vi "VersionController.vi"() -> ()   [LabVIEW 2019, in "ByteLVDevEnv.lvlib"]
uses:
  ByteLVDevEnv.lvlib
  TypeDefs/LibraryVersions.ctl
  TypeDefs/AllLibraries.ctl
  <vilib>/regexp/Match Regular Expression.xnode
  <vilib>/JKI/VIPM API/VIPM API_vipm_api.lvlib
panel:
  in  "Select Labview Version":u16(ring) items=["19.0"]
  out "Status":string
  in  "Exit":bool
  in  "Restart":bool
  out "LOADING":string
  out "packets.txt errors":string[](array[string])
  in  "Local VIP Folder":path
  out "VIP files found in local folder":string
  out "Install log":string[](array[string])
  in  "Start":bool
  in  "packets.txt Path":path
  # "VIP Package Installer"
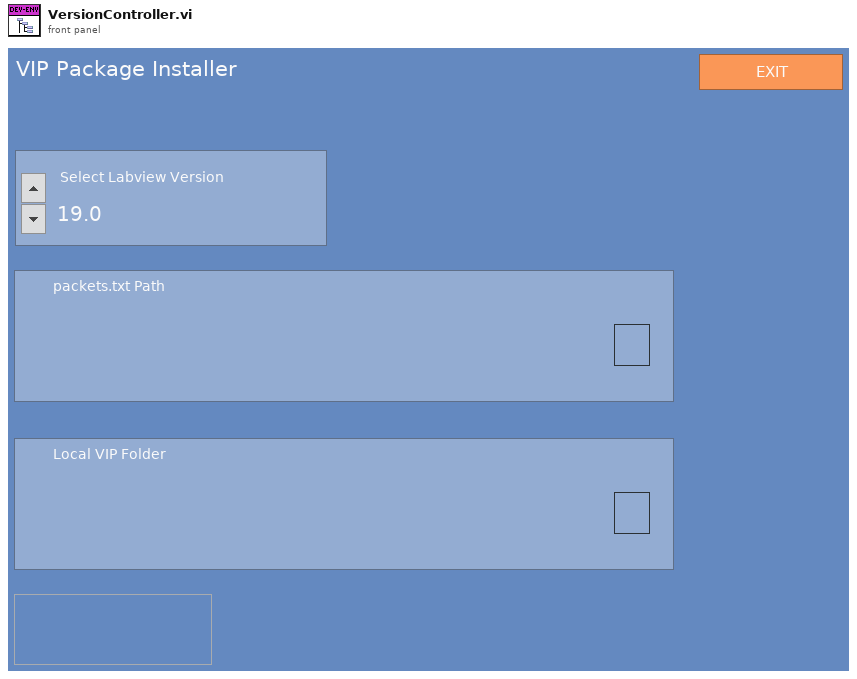
[diagram p1: front panel]
types:
  T1 = typedef "ByteLVDevEnv.lvlib/AllLibraries.ctl" = cluster{"Package Name":string, "Version":string, "Installed":bool, "Path":path}
  T2 = typedef "ByteLVDevEnv.lvlib/LibraryVersions.ctl" = cluster{"Name":string, "Version 1 ":string, "Version 2":string, "Sign 1":string, "Sign 2":string, "Function":string, "V. Install":string}
  T3 = cluster{"LOADING":refnum<vi>, "Local VIP Folder":refnum<vi>, "packets.txt Path ":refnum<vi>, "Start":refnum<vi>, "Install log":refnum<vi>, "VIP files found in local folder":refnum<vi>, "packets.txt errors":refnum<vi>, "Restart":refnum<vi>, "Exit":refnum<vi>, "Status":refnum<vi>, "Select Labview Version":refnum<vi>}
  T4 = cluster{"Status":string, "Versions":T2[], "All Packages":T1[], "LabView V.":string, "LocalVip":T1[], "Log":string[], "Packets errors":string[]}
  T5 = enum8{"Enabled", "Disabled", "Disabled and Grayed Out"}
  T6 = enum16{"open", "replace", "create", "open or create", "replace or create", "replace or create with confirmation"}
  T7 = cluster{"packets.txt Path ":path, "Local VIP Folder":path, "Select Labview Version":u16}
  T8 = typedef "VIPM API_vipm_api.lvlib/LabVIEW Target Info Cluster_vipm_api.ctl" = cluster{"Version":string, "Connection Tested":bool, "Disabled":bool}
  T9 = typedef "LVStringsAndValuesArrayTypeDef_U16.ctl" = cluster{"String":string, "Value":u16}[]
  T10 = typedef "VIPM API_vipm_api.lvlib/Library Contents Cluster_vipm_api.ctl" = cluster{"Package Name":string, "Version":string, "Display Name":string, "Repository Name":string, "Company Name":string, "License Type":string, "Installed":bool, "Deprecated":bool, "Dependency or Conflict Problem":bool, "Downloaded":bool}
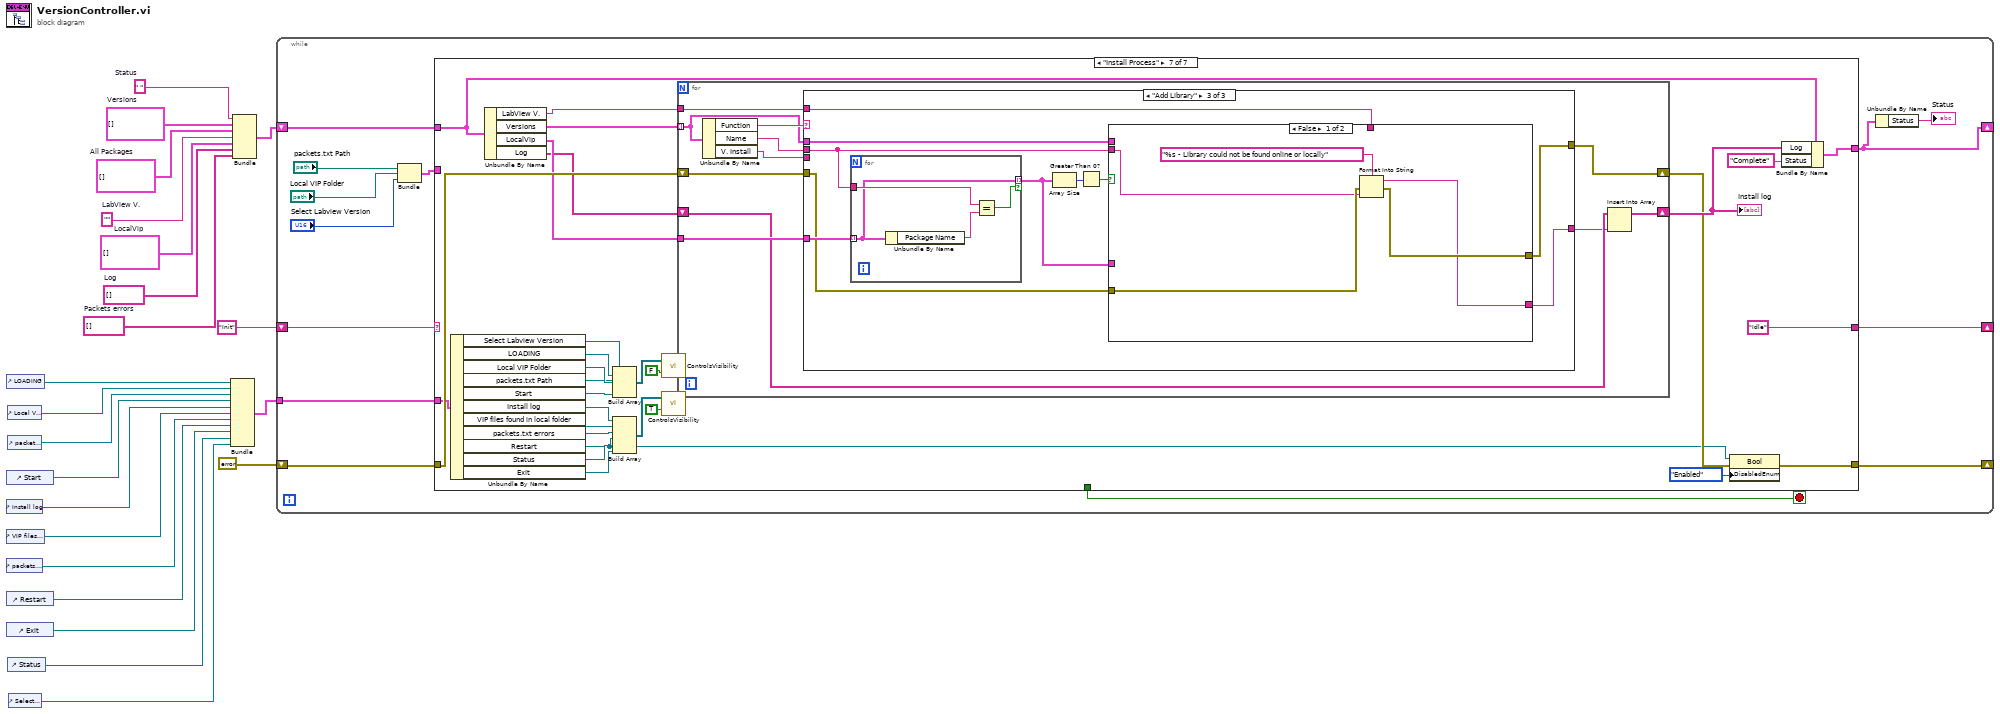
[diagram p0: block diagram]
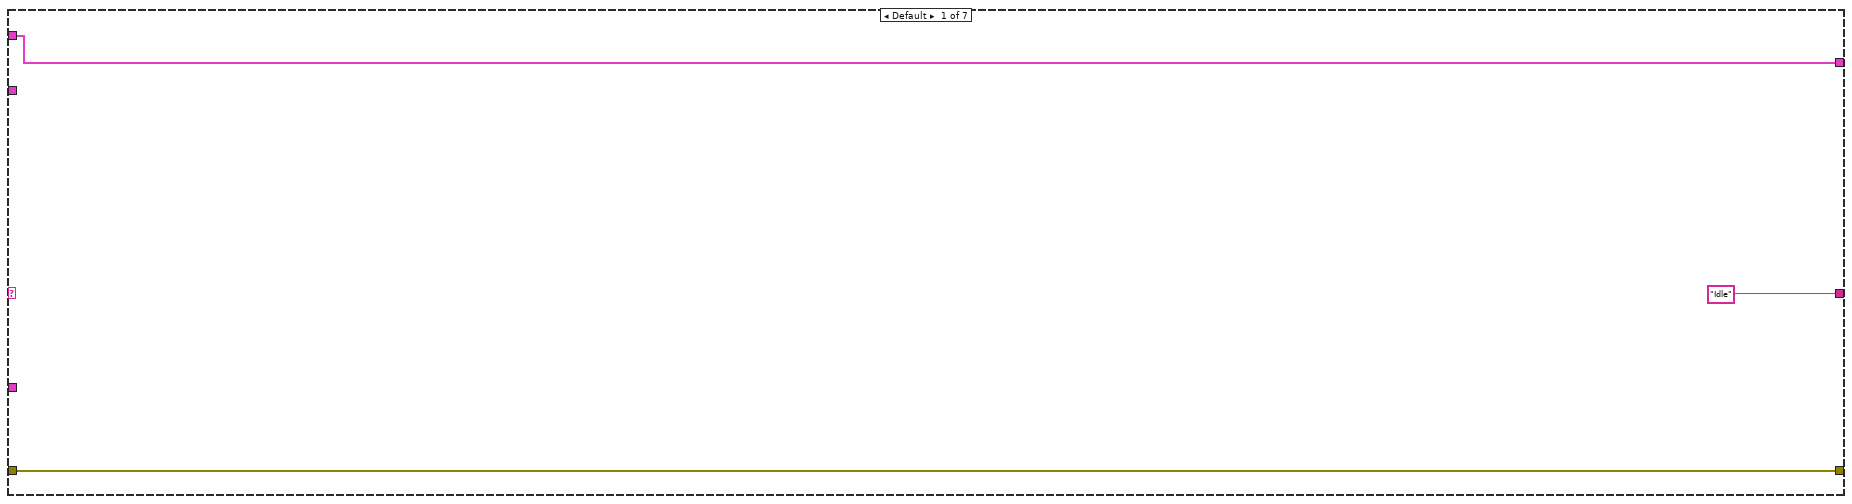
[diagram p2: hidden frame]
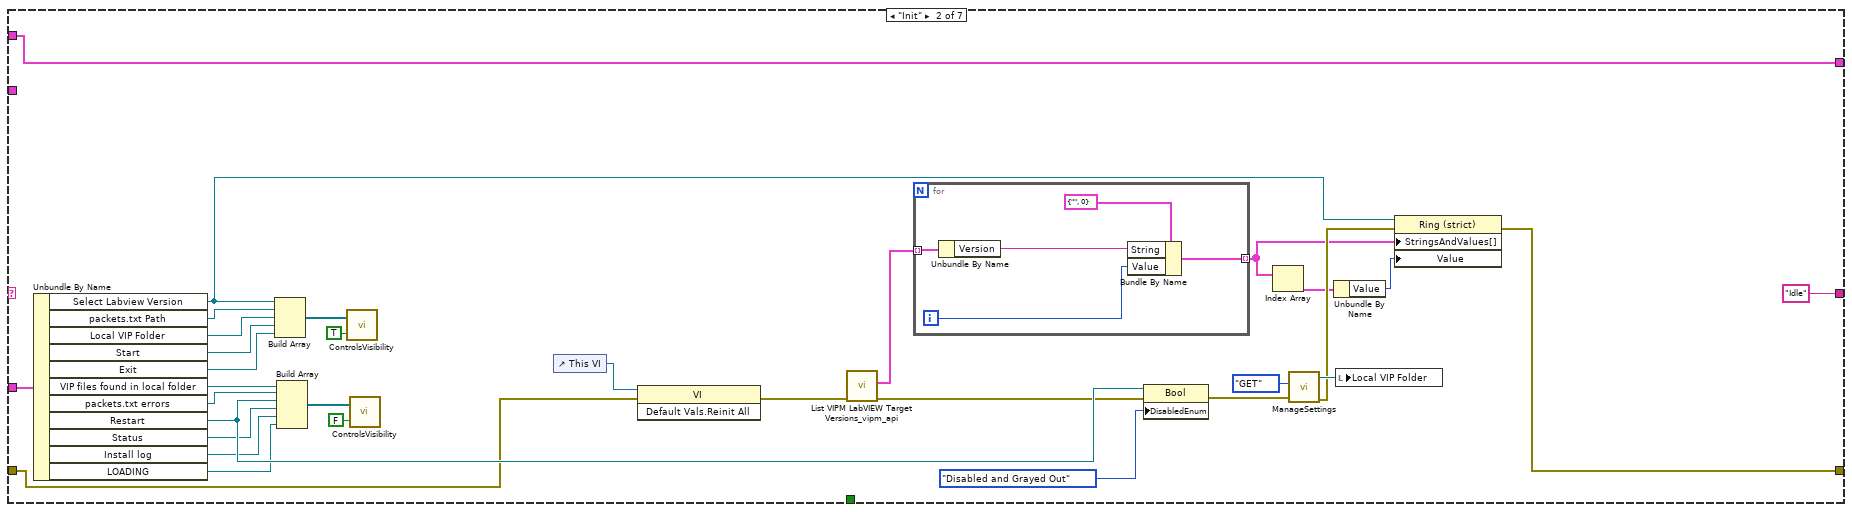
[diagram p3: hidden frame]
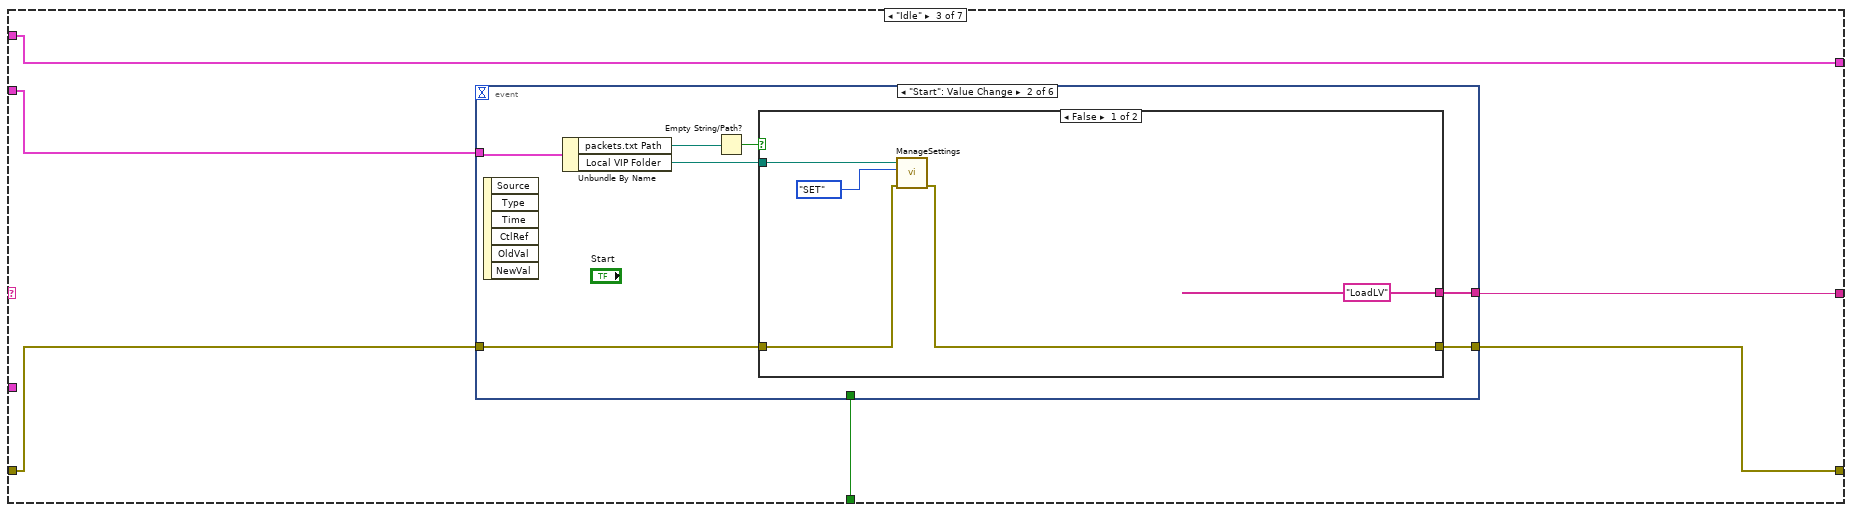
[diagram p4: hidden frame]
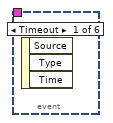
[diagram p5: hidden frame]
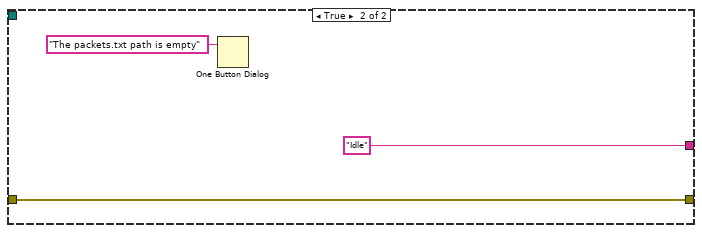
[diagram p6: hidden frame]
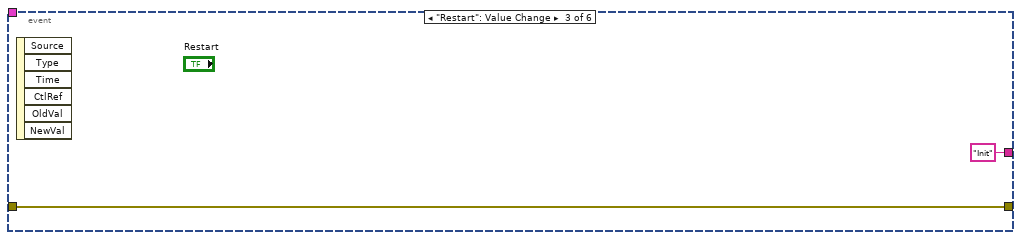
[diagram p7: hidden frame]
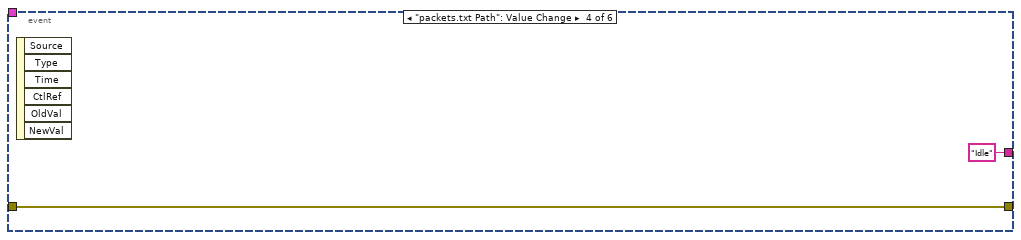
[diagram p8: hidden frame]
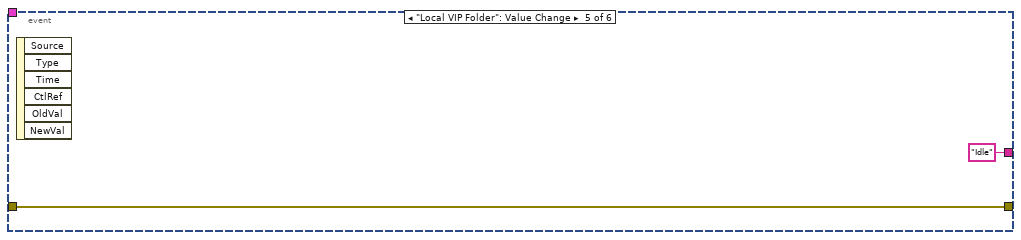
[diagram p9: hidden frame]
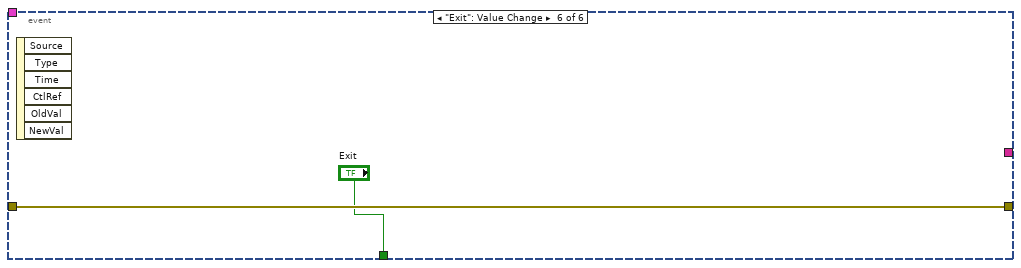
[diagram p10: hidden frame]
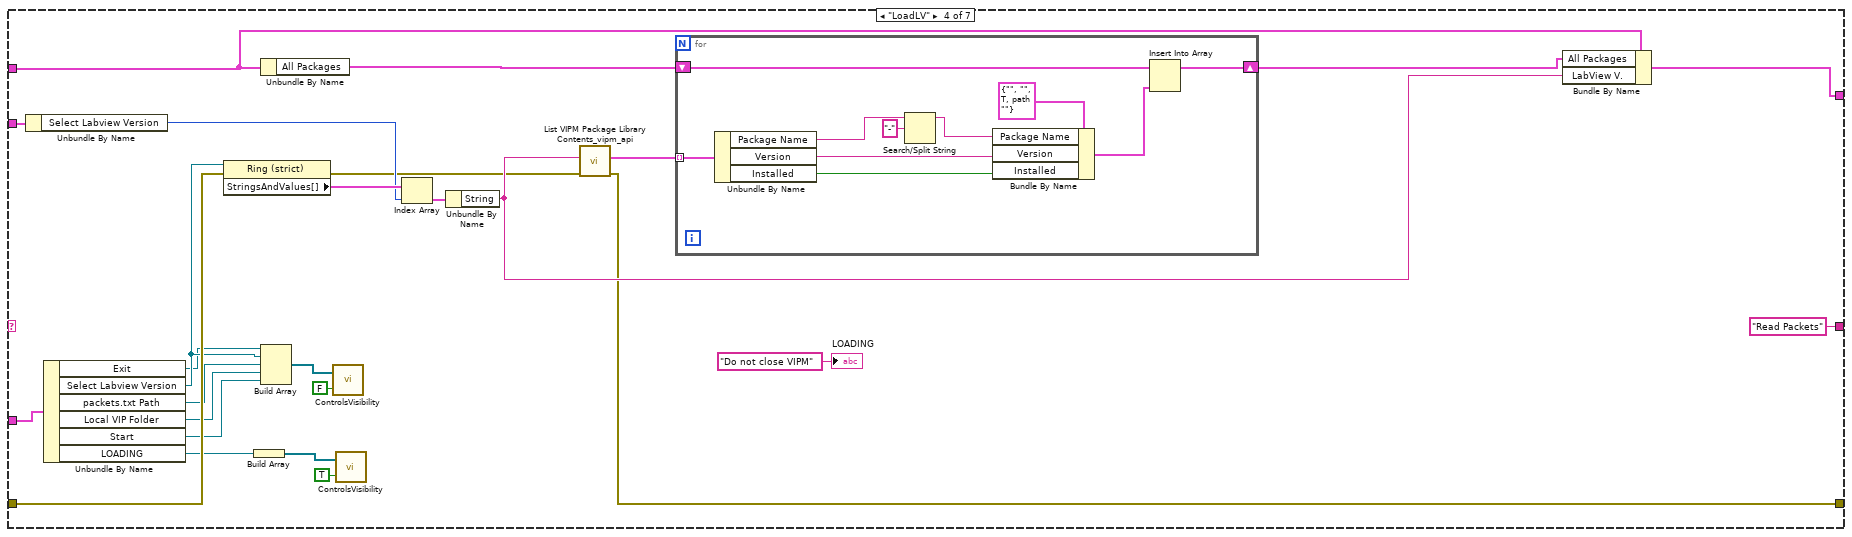
[diagram p11: hidden frame]
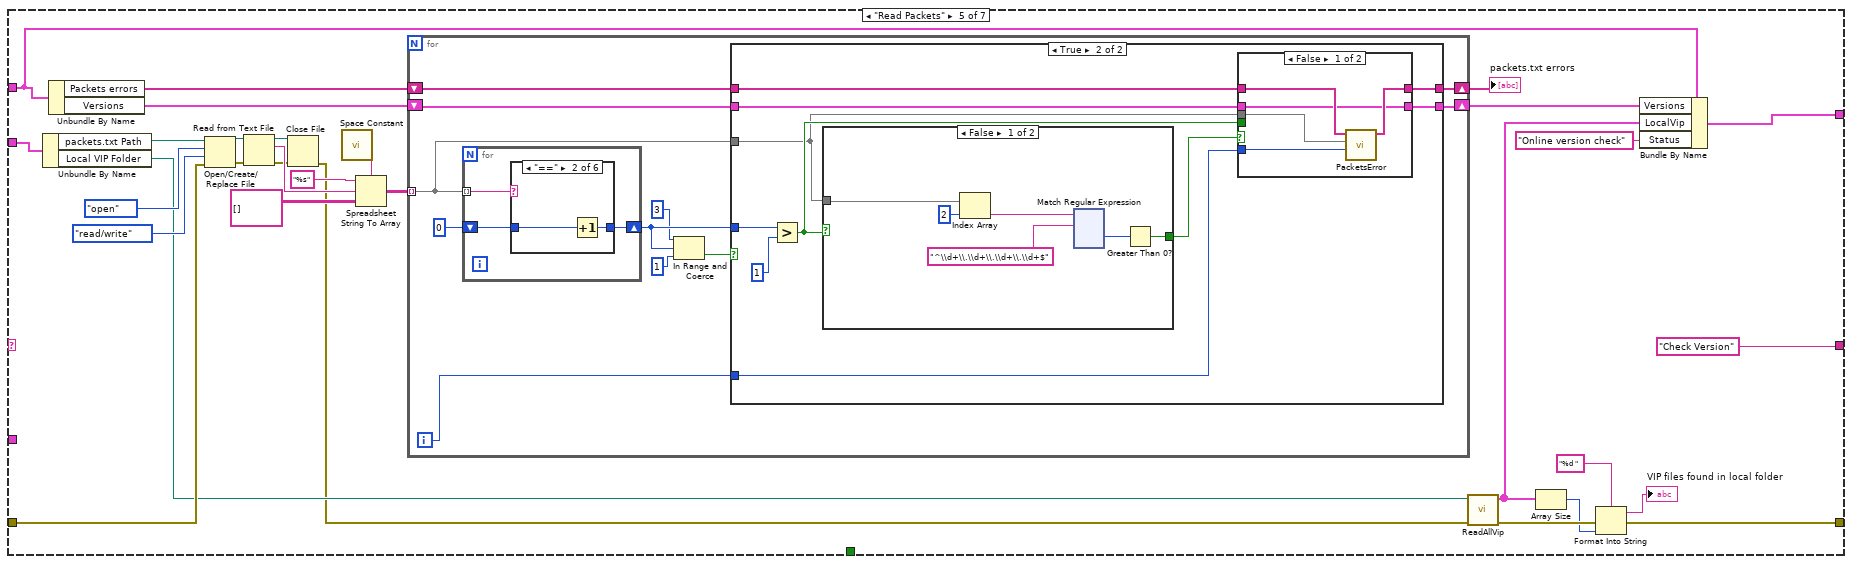
[diagram p12: hidden frame]
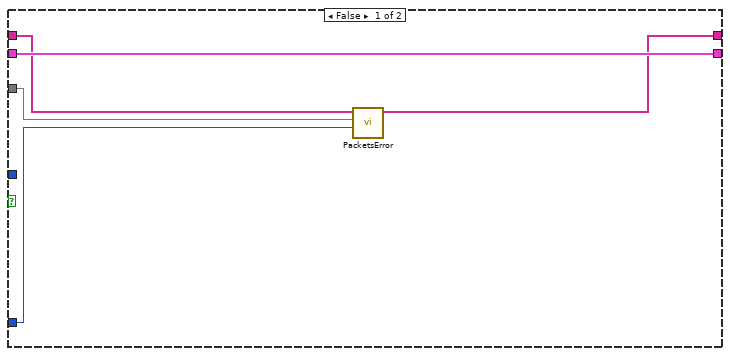
[diagram p13: hidden frame]
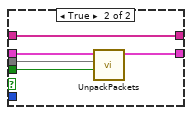
[diagram p14: hidden frame]
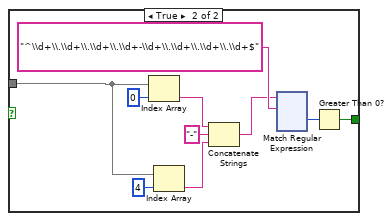
[diagram p15: hidden frame]
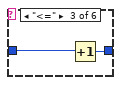
[diagram p17: hidden frame]
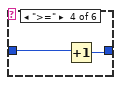
[diagram p18: hidden frame]
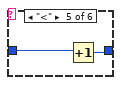
[diagram p19: hidden frame]
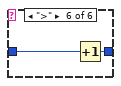
[diagram p20: hidden frame]
diagram:
  w3 = " "  # Status
  w14 = string[] []  # Packets errors
  w15 = string[] []  # Log
  w16 = T1[] []  # LocalVip
  w18 = ""  # LabView V.
  w19 = T1[] []  # All Packages
  w21 = T2[] []  # Versions
  n1 = control-ref of="LOADING"() -> (w13:refnum<vi>)
  n2 = control-ref of="Start"() -> (w10:refnum<vi>)
  n3 = control-ref of="Install log"() -> (w9:refnum<vi>)
  n4 = control-ref of="VIP files found in local folder"() -> (w8:refnum<vi>)
  n5 = control-ref of="packets.txt errors"() -> (w7:refnum<vi>)
  n6 = control-ref of="Restart"() -> (w5:refnum<vi>)
  n7 = control-ref of="Exit"() -> (w4:refnum<vi>)
  n8 = control-ref of="Local VIP Folder"() -> (w12:refnum<vi>)
  n9 = control-ref of="packets.txt Path"() -> (w11:refnum<vi>)
  n10 = control-ref of="Status"() -> (w2:refnum<vi>)
  n11 = control-ref of="Select Labview Version"() -> (w1:refnum<vi>)
  n12 = Bundle("LOADING"=w13, "Local VIP Folder"=w12, "packets.txt Path"=w11, "Start"=w10, "Install log"=w9, "VIP files found in local folder"=w8, "packets.txt errors"=w7, "Restart"=w5, "Exit"=w4, "Status"=w2, "Select Labview Version"=w1) -> (w6:T3)  [unwired: 1 in]
  n13 = Bundle("Status"=w3, "Versions"=w21, "All Packages"=w19, "LabView V."=w18, "LocalVip"=w16, "Log"=w15, "Packets errors"=w14) -> (w20:T4)  [unwired: 1 in]
  n14 = while {
    shift-right: [w32] -> _
    shift-left: "Init" -> [w35]
    shift-right: [w25] -> _
    shift-left: w20 -> [w31]
    shift-right: [w30] -> _
    shift-left: errorcluster {"status"=FALSE, "code"=0, "source"=""} ("error in") -> [w29]
    tunnel: w6 -> [w27]
    stop <- w26 stop-if-true
    n15 = Bundle("packets.txt Path"="packets.txt Path", "Local VIP Folder"="Local VIP Folder", "Select Labview Version"="Select Labview Version") -> (w33:T7)  [unwired: 1 in]
    n16 = case shown="\"Install Process\"" w35 {
      tunnel: w33 -> [_ _ w79 w122 w170 _ _]
      tunnel: ["Idle" "Idle" w81 "Read Packets" "Check Version" "Install Process" "Idle"] -> w32
      tunnel: w31 -> [w37 w69 w80 w128 w157 w469 w519]
      tunnel: w29 -> [w36 w48 w78 w124 w168 w470 w523]
      tunnel: [w37 w69 w80 w127 w155 w466 w518] -> w25
      tunnel: [w36 w43 w77 w107 w148 w470 w502] -> w30
      tunnel: w27 -> [_ w65 _ w125 _ _ w506]
      tunnel: [_ _ w76 _ _ _ _] -> w26
      frame Default {
      }
      frame "Init" {
        n17 = Unbundle By Name(w65) -> ("Select Labview Version"=w42:refnum<vi>, "packets.txt Path"=w60:refnum<vi>, "Local VIP Folder"=w59:refnum<vi>, "Start"=w58:refnum<vi>, "Exit"=w57:refnum<vi>, "VIP files found in local folder"=w56:refnum<vi>, "packets.txt errors"=w55:refnum<vi>, "Restart"=w54:refnum<vi>, "Status"=w53:refnum<vi>, "Install log"=w52:refnum<vi>, "LOADING"=w51:refnum<vi>)
        n18 = Build Array(w42, w60, w59, w58, w57) -> (w49:refnum<vi>[])
        n19 = Build Array(w56, w55, w54, w53, w52, w51) -> (w50:refnum<vi>[])
        n20 = call "ControlsVisibility.vi"("Visible"=TRUE, "Array"=w49) -> ()  [unwired: 2 in]
        n21 = call "ControlsVisibility.vi"("Visible"=FALSE, "Array"=w50) -> ()  [unwired: 2 in]
        n22 = control-ref of="This VI"() -> (w67:refnum<vi>)
        n23 = invoke class="VI" method="Default Vals.Reinit All"(reference=w67, error in=w48) -> (error out=w47:errorcluster)  [unwired: 1 in, 2 out]
        n24 = call <vilib>:"List VIPM LabVIEW Target Versions_vipm_api.vi"("error in (no error)"=w47) -> ("error out"=w46:errorcluster, "LabVIEW Target Info"=w45:T8[])  [unwired: 9 in]
        n25 = for {
          tunnel: w45 -> [w74] mode=indexing
          tunnel: [w71] -> w41 mode=indexing
          i -> [w72]
          n26 = Unbundle By Name(w74) -> ("Version"=w73:string)
          n27 = Bundle By Name(cluster=cluster{"String":string, "Value":u16} {"String"="", "Value"=0} ("Cluster"), "String"=w73, "Value"=w72) -> (w71:cluster{"String":string, "Value":u16})
        }
        n28 = property class="Bool"(reference=w54, error in=w46, "DisabledEnum"=T5."Disabled and Grayed Out" ("Disabled")) -> (error out=w63:errorcluster)  [unwired: 1 out]
        n29 = Index Array(array=w41) -> (element=w40:cluster{"String":string, "Value":u16})  [unwired: 1 in]
        n30 = call "ManageSettings.vi"("error in (no error)"=w63, "Mode"=enum16{"GET", "SET"}."GET") -> ("error out"=w44:errorcluster, "File Path Out"=w66:path)  [unwired: 8 in]
        n31 = Unbundle By Name(w40) -> ("Value"=w39:u16)
        n32 = local write "Local VIP Folder"(w66) -> ()
        n33 = property class="Ring (strict)"(reference=w42, error in=w44, "StringsAndValues[]"=w41, "Value"=w39) -> (error out=w43:errorcluster)  [unwired: 1 out]
      }
      frame "Idle" {
        n34 = event shown="[1] \"Start\": Value Change" {
          selector: _ -> [_ _ _ _ _ _]
          dyn-events: _ -> [_ _ _ _ _ _]
          timeout: _ -> [_ _ _ _ _ _]
          tunnel: [_ w85 "Init" "Idle" "Idle" _] -> w81
          tunnel: w79 -> [_ w88 _ _ _ _]
          tunnel: w78 -> [_ w83 w98 w99 w101 w104]
          tunnel: [_ w82 w98 w99 w101 w104] -> w77
          tunnel: [_ _ _ _ _ "Exit"] -> w76
          event Timeout {
            n35 = event-data() -> ()  [unwired: 1 in, 3 out]
          }
          event "Start": Value Change {
            n36 = event-data() -> ()  [unwired: 1 in, 6 out]
            n37 = Unbundle By Name(w88) -> ("packets.txt Path"=w87:path, "Local VIP Folder"=w84:path)
            n38 = Empty String/Path?(string/path=w87) -> (empty?=w86:bool)
            n39 = case shown="False" w86 {
              tunnel: ["LoadLV" "Idle"] -> w85
              tunnel: w84 -> [w92 _]
              tunnel: w83 -> [w90 w95]
              tunnel: [w89 w95] -> w82
              frame False {
                n40 = call "ManageSettings.vi"("error in (no error)"=w90, "Mode"=enum16{"GET", "SET"}."SET", "File Path"=w92) -> ("error out"=w89:errorcluster)  [unwired: 7 in, 1 out]
              }
              frame True {
                n41 = One Button Dialog(message="The packets.txt path is empty") -> ()  [unwired: 1 in, 1 out]
              }
            }
          }
          event "Restart": Value Change {
            n42 = event-data() -> ()  [unwired: 1 in, 6 out]
          }
          event "packets.txt Path": Value Change {
            n43 = event-data() -> ()  [unwired: 1 in, 6 out]
          }
          event "Local VIP Folder": Value Change {
            n44 = event-data() -> ()  [unwired: 1 in, 6 out]
          }
          event "Exit": Value Change {
            n45 = event-data() -> ()  [unwired: 1 in, 6 out]
          }
        }
      }
      frame "LoadLV" {
        n46 = Unbundle By Name(w122) -> ("Select Labview Version"=w121:u16)
        n47 = Unbundle By Name(w125) -> ("Exit"=w105:refnum<vi>, "Select Labview Version"=w112:refnum<vi>, "packets.txt Path"=w111:refnum<vi>, "Local VIP Folder"=w110:refnum<vi>, "Start"=w109:refnum<vi>, "LOADING"=w108:refnum<vi>)
        n48 = property class="Ring (strict)"(reference=w112, error in=w124) -> (error out=w117:errorcluster, "StringsAndValues[]"=w123:T9)  [unwired: 1 out]
        n49 = Build Array(w108) -> (w114:refnum<vi>[])
        n50 = Unbundle By Name(w128) -> ("All Packages"=w130:T1[])
        n51 = Build Array(w105, w112, w111, w110, w109) -> (w113:refnum<vi>[])
        n52 = call "ControlsVisibility.vi"("Visible"=FALSE, "Array"=w113) -> ()  [unwired: 2 in]
        n53 = call "ControlsVisibility.vi"("Visible"=TRUE, "Array"=w114) -> ()  [unwired: 2 in]
        n54 = Index Array(array=w123, index=w121) -> (element=w120:cluster{"String":string, "Value":u16})
        n55 = Unbundle By Name(w120) -> ("String"=w119:string)
        n56 = call <vilib>:"List VIPM Package Library Contents_vipm_api.vi"("error in (no error)"=w117, "LabVIEW Version"=w119) -> ("error out"=w107:errorcluster, "Library Contents []"=w129:T10[])  [unwired: 7 in, 1 out]
        n57 = for {
          tunnel: w129 -> [w140] mode=indexing
          shift-right: [w133] -> w126
          shift-left: w130 -> [w132]
          n58 = Unbundle By Name(w140) -> ("Package Name"=w138:string, "Version"=w135:string, "Installed"=w134:bool)
          n59 = Search/Split String(string=w138, search string/char (-)="-") -> (substring before match=w136:string)  [unwired: 1 in, 2 out]
          n60 = Bundle By Name(cluster=T1 {"Package Name"="", "Version"="", "Installed"=TRUE, "Path"=path ""}, "Package Name"=w136, "Version"=w135, "Installed"=w134) -> (w131:T1)
          n61 = Insert Into Array(array=w132, new element=w131) -> (w133:T1[])  [unwired: 1 in]
        }
        n62 = Bundle By Name(cluster=w128, "All Packages"=w126, "LabView V."=w119) -> (w127:T4)
        "LOADING" <- "Do not close VIPM" ("LOADING")
      }
      frame "Read Packets" {
        n63 = Unbundle By Name(w170) -> ("packets.txt Path"=w169:path, "Local VIP Folder"=w153:path)
        n64 = Unbundle By Name(w157) -> ("Packets errors"=w146:string[], "Versions"=w158:T2[])
        n65 = Open/Create/Replace File(file path (use dialog)=w169, error in=w168, operation (0:open)=T6."open", access (0:read/write)=enum16{"read/write", "read-only", "write-only"}."read/write") -> (refnum out=w165:refnum<file>, error out=w164:errorcluster)  [unwired: 2 in, 1 out]
        n66 = Read from Text File(file (use dialog)=w165, error in=w164) -> (refnum out=w142:refnum<file>, text=w163:string, error out=w143:errorcluster)  [unwired: 2 in, 1 out]
        n67 = Close File(refnum=w142, error in=w143) -> (error out=w141:errorcluster)  [unwired: 1 out]
        n68 = call <vilib>:"Space Constant.vi"() -> ("String"=w159:string)
        n69 = Spreadsheet String To Array(delimiter (Tab)=w159, format string="%s", spreadsheet string=w163, array type (2D Dbl)=string[][] []) -> (array=w160:string[][])
        n70 = for {
          tunnel: w160 -> [w178] mode=indexing
          shift-right: [w180] -> w156
          shift-left: w158 -> [w181]
          shift-right: [w172] -> w145
          shift-left: w146 -> [w173]
          i -> [w171]
          n71 = for {
            tunnel: w178 -> [w453] mode=indexing
            shift-right: [w451] -> w177
            shift-left: 0 -> [w452]
            n72 = case shown="\"==\"" w453 {
              tunnel: w452 -> [w454 w456 w458 w460 w462 w464]
              tunnel: [w454 w455 w457 w459 w461 w463] -> w451
              frame Default {
              }
              frame "==" {
                n73 = Increment(x=w456) -> (x+1=w455:i32)
              }
              frame "<=" {
                n74 = Increment(x=w458) -> (x+1=w457:i32)
              }
              frame ">=" {
                n75 = Increment(x=w460) -> (x+1=w459:i32)
              }
              frame "<" {
                n76 = Increment(x=w462) -> (x+1=w461:i32)
              }
              frame ">" {
                n77 = Increment(x=w464) -> (x+1=w463:i32)
              }
            }
          }
          n78 = In Range and Coerce(upper limit=3, x=w177, lower limit=1) -> (In Range?=w174:bool)  [unwired: 1 out]
          n79 = case shown="True" w174 {
            tunnel: w181 -> [w186 w196]
            tunnel: [w186 w195] -> w180
            tunnel: w178 -> [w185 w191]
            tunnel: w177 -> [_ w193]
            tunnel: w173 -> [w184 w190]
            tunnel: [w183 w189] -> w172
            tunnel: w171 -> [w182 w188]
            frame False {
              n80 = call "PacketsError.vi"("Index"=w182, "Libraries"=w185, "Packets errors in"=w184) -> ("Packets errors out"=w183:string[])  [unwired: 8 in]
            }
            frame True {
              n81 = Greater?(x=w193, y=1) -> (0:w192:bool)
              n82 = case shown="False" w192 {
                tunnel: w191 -> [w212 w332]
                tunnel: [w208 w331] -> w187
                frame False {
                  n83 = Index Array(array=w212, index=2) -> (element=w210:string)
                  n84 = xnode "Match Regular Expression"("input string"=w210, "regular expression"="^\\d+\\.\\d+\\.\\d+\\.\\d+$") -> ("offset past match"=w207:i32)  [unwired: 4 in, 4 out]
                  n85 = Greater Than 0?(x=w207) -> (x > 0?=w208:bool)
                }
                frame True {
                  n86 = Index Array(array=w332, index=0) -> (element=w330:string)
                  n87 = Index Array(array=w332, index=4) -> (element=w329:string)
                  n88 = Concatenate Strings(w330, "-" ("string"), w329) -> (w327:string)
                  n89 = xnode "Match Regular Expression"("input string"=w327, "regular expression"="^\\d+\\.\\d+\\.\\d+\\.\\d+-\\d+\\.\\d+\\.\\d+\\.\\d+$") -> ("offset past match"=w334:i32)  [unwired: 4 in, 4 out]
                  n90 = Greater Than 0?(x=w334) -> (x > 0?=w331:bool)
                }
              }
              n91 = case shown="False" w187 {
                tunnel: w196 -> [w198 w206]
                tunnel: [w198 w205] -> w195
                tunnel: w192 -> [_ w204]
                tunnel: w191 -> [w197 w203]
                tunnel: w190 -> [w200 w202]
                tunnel: [w199 w202] -> w189
                tunnel: w188 -> [w201 _]
                frame False {
                  n92 = call "PacketsError.vi"("Index"=w201, "Libraries"=w197, "Packets errors in"=w200) -> ("Packets errors out"=w199:string[])  [unwired: 8 in]
                }
                frame True {
                  n93 = call "UnpackPackets.vi"("Type"=w204, "Libraries"=w203, "Versions in"=w206) -> ("Versions out"=w205:T2[])  [unwired: 8 in]
                }
              }
            }
          }
        }
        "packets.txt errors" <- w145
        n94 = call "ReadAllVip.vi"("error in (no error)"=w141, "Cartella VIP locale"=w153) -> ("error out"=w151:errorcluster, "LocalVip"=w152:T1[])  [unwired: 8 in]
        n95 = Array Size(array=w152) -> (size(s)=w150:i32)
        n96 = Format Into String(format string="%d ", error in=w151, w150) -> (resulting string=→"VIP files found in local folder":string, error out=w148:errorcluster)  [unwired: 1 in]
        n97 = Bundle By Name(cluster=w157, "Versions"=w156, "LocalVip"=w152, "Status"="Online version check") -> (w155:T4)
      }
      frame "Check Version" {
        n98 = Unbundle By Name(w469) -> ("Versions"=w468:T2[], "All Packages"=w471:T1[])
        n99 = for {
          tunnel: w468 -> [w477] mode=indexing
          tunnel: w471 -> [w482]
          shift-right: [w473] -> w467
          shift-left: w468 -> [w474]
          i -> [w476]
          n100 = Unbundle By Name(w477) -> ("Name"=w481:string)
          n101 = for {
            tunnel: w482 -> [w494] mode=indexing
            tunnel: w481 -> [w495]
            tunnel: [w494] -> w478 mode=indexing if=w493
            n102 = Unbundle By Name(w494) -> ("Package Name"=w496:string)
            n103 = Equal?(x=w495, y=w496) -> (x = y?=w493:bool)
          }
          n104 = Array Size(array=w478) -> (size(s)=w480:i32)
          n105 = Greater Than 0?(x=w480) -> (x > 0?=w479:bool)
          n106 = case shown="True" w479 {
            tunnel: w478 -> [_ w491]
            tunnel: w477 -> [w485 w490]
            tunnel: [w483 w492] -> w475
            frame False {
              n107 = Bundle By Name(cluster=w485, "Function"="Add Library") -> (w483:T2)
            }
            frame True {
              n108 = call "CheckVersion.vi"("Array"=w491, "Cluster in"=w490) -> ("Checkbox"=w488:bool, "Cluster out"=w489:T1)  [unwired: 8 in]
              n109 = call "SelectFunction.vi"("Found?"=w488, "Library"=w489) -> ("Version"=w486:string, "Function"=w487:string)  [unwired: 8 in]
              n110 = Bundle By Name(cluster=w490, "Function"=w487, "V. Install"=w486) -> (w492:T2)
            }
          }
          n111 = Replace Array Subset(array=w474, new element=w475, index=w476) -> (w473:T2[])
        }
        n112 = Bundle By Name(cluster=w469, "Versions"=w467, "Status"="Installing") -> (w466:T4)
      }
      frame "Install Process" {
        n113 = Unbundle By Name(w506) -> ("Select Labview Version"=w498:refnum<vi>, "LOADING"=w499:refnum<vi>, "Local VIP Folder"=w516:refnum<vi>, "packets.txt Path"=w515:refnum<vi>, "Start"=w514:refnum<vi>, "Install log"=w511:refnum<vi>, "VIP files found in local folder"=w510:refnum<vi>, "packets.txt errors"=w509:refnum<vi>, "Restart"=w501:refnum<vi>, "Status"=w504:refnum<vi>, "Exit"=w497:refnum<vi>)
        n114 = Unbundle By Name(w519) -> ("LabView V."=w522:string, "Versions"=w524:T2[], "LocalVip"=w521:T1[], "Log"=w520:string[])
        n115 = Build Array(w498, w499, w516, w515, w514) -> (w508:refnum<vi>[])
        n116 = Build Array(w511, w510, w509, w501, w504, w497) -> (w507:refnum<vi>[])
        n117 = call "ControlsVisibility.vi"("Visible"=FALSE, "Array"=w508) -> ()  [unwired: 2 in]
        n118 = call "ControlsVisibility.vi"("Visible"=TRUE, "Array"=w507) -> ()  [unwired: 2 in]
        n119 = for {
          tunnel: w524 -> [w529] mode=indexing
          shift-right: [w531] -> w503
          shift-left: w523 -> [w535]
          tunnel: w522 -> [w532]
          tunnel: w521 -> [w530]
          shift-right: [w526] -> w517
          shift-left: w520 -> [w528]
          n120 = Unbundle By Name(w529) -> ("Function"=w536:string, "Name"=w534:string, "V. Install"=w533:string)
          n121 = case shown="\"Add Library\"" w536 {
            tunnel: w535 -> [w542 w553 w559]
            tunnel: w534 -> [w538 w551 w555]
            tunnel: w533 -> [w537 w550 _]
            tunnel: w532 -> [_ w548 w557]
            tunnel: [w541 w544 w558] -> w531
            tunnel: w530 -> [_ _ w561]
            tunnel: w529 -> [_ _ w560]
            tunnel: [w539 w543 w556] -> w527
            frame "Skip", Default {
              n122 = Format Into String(format string="%s-%s - Library already installed", error in=w542, w538, w537) -> (resulting string=w539:string, error out=w541:errorcluster)  [unwired: 1 in]
            }
            frame "Install" {
              n123 = Format Into String(format string="%s-%s", error in=w553, w551, w550) -> (resulting string=w545:string, error out=w552:errorcluster)  [unwired: 1 in]
              n124 = Build Array(w545) -> (w549:string[])
              n125 = call <vilib>:"Install VI Packages by Name_vipm_api.vi"("error in (no error)"=w552, "LabVIEW Version"=w548, "Package Names to Install []"=w549) -> ("error out"=w546:errorcluster)  [unwired: 8 in]
              n126 = Format Into String(format string="%s - Installed From VIPM Library", error in=w546, w545) -> (resulting string=w543:string, error out=w544:errorcluster)  [unwired: 1 in]
            }
            frame "Add Library" {
              n127 = for {
                tunnel: w561 -> [w598] mode=indexing
                tunnel: w555 -> [w599]
                tunnel: [w598] -> w562 mode=indexing if=w597
                n128 = Unbundle By Name(w598) -> ("Package Name"=w600:string)
                n129 = Equal?(x=w599, y=w600) -> (x = y?=w597:bool)
              }
              n130 = Array Size(array=w562) -> (size(s)=w564:i32)
              n131 = Greater Than 0?(x=w564) -> (x > 0?=w563:bool)
              n132 = case shown="False" w563 {
                tunnel: w562 -> [_ w578]
                tunnel: w560 -> [_ w577]
                tunnel: w559 -> [w569 w574]
                tunnel: [w568 w573] -> w558
                tunnel: w557 -> [_ w572]
                tunnel: [w566 w571] -> w556
                tunnel: w555 -> [w565 w570]
                frame False {
                  n133 = Format Into String(format string="%s - Library could not be found online or locally", error in=w569, w565) -> (resulting string=w566:string, error out=w568:errorcluster)  [unwired: 1 in]
                }
                frame True {
                  n134 = call "CheckVersion.vi"("Array"=w578, "Cluster in"=w577) -> ("Checkbox"=w576:bool, "Cluster out"=w575:T1)  [unwired: 8 in]
                  n135 = case shown="True" w576 {
                    tunnel: w575 -> [_ w596]
                    tunnel: w574 -> [w582 w591]
                    tunnel: [w581 w588] -> w573
                    tunnel: w572 -> [_ w590]
                    tunnel: [w580 w584] -> w571
                    tunnel: w570 -> [w579 _]
                    frame False {
                      n136 = Format Into String(format string="%s - Version of Library could not be found online or locally", error in=w582, w579) -> (resulting string=w580:string, error out=w581:errorcluster)  [unwired: 1 in]
                    }
                    frame True {
                      n137 = Unbundle By Name(w596) -> ("Package Name"=w586:string, "Version"=w585:string, "Path"=w595:path)
                      n138 = Build Array(w595) -> (w594:path[])
                      n139 = call <vilib>:"Add VI Packages to VIPM Package Library_vipm_api.vi"("error in (no error)"=w591, "Packages to add to VIPM Library (vipc,vip,ogp)"=w594) -> ("error out"=w593:errorcluster, "Package Names Added"=w592:string[])  [unwired: 8 in]
                      n140 = call <vilib>:"Install VI Packages by Name_vipm_api.vi"("error in (no error)"=w593, "LabVIEW Version"=w590, "Package Names to Install []"=w592) -> ("error out"=w589:errorcluster)  [unwired: 8 in]
                      n141 = Format Into String(format string="%s-%s - Installed from local folder", error in=w589, w586, w585) -> (resulting string=w584:string, error out=w588:errorcluster)  [unwired: 1 in]
                    }
                  }
                }
              }
            }
          }
          n142 = Insert Into Array(array=w528, new element=w527) -> (w526:string[])  [unwired: 1 in]
        }
        "Install log" <- w517
        n143 = property class="Bool"(reference=w501, error in=w503, "DisabledEnum"=T5."Enabled" ("Disabled")) -> (error out=w502:errorcluster)  [unwired: 1 out]
        n144 = Bundle By Name(cluster=w519, "Log"=w517, "Status"="Complete") -> (w518:T4)
      }
    }
    n145 = Unbundle By Name(w25) -> ("Status"=→"Status":string)
  }
